vi "Stop.vi"(8 "error in (no error)":errorcluster, 11 "RIO_API in":refnum<class "9770 API.lvclass">) -> (0 "error out":errorcluster, 3 "RIO_API out":refnum<class "9770 API.lvclass">)   [LabVIEW 2017, in "9770 API.lvclass"]
uses:
  <vilib>/addons/InsightCM/Devices/Shared/Emsa/Emsa9770API/9770 API.lvclass
  <vilib>/addons/InsightCM/Devices/Shared/Emsa/Emsa9770API/9770 API.lvclass/9770 API.ctl
  <vilib>/Utility/error.llb/Error Cluster From Error Code.vi
  <vilib>/rvi/errors/niLvFpgaAdjustHostInterfaceError.vi
  <vilib>/ErrorRing/Error Ring.xnode
  <vilib>/rvi/interface/nirviReadWriteControl/nirviReadWriteControl.xnode
  <vilib>/addons/InsightCM/Devices/Shared/Emsa/Emsa9770API/controls/FPGATypeDef.ctl
  NiFpgaLv.dll
  <vilib>/rvi/interface/Simulation/niFpgaSimulationCallBeginRW.vi
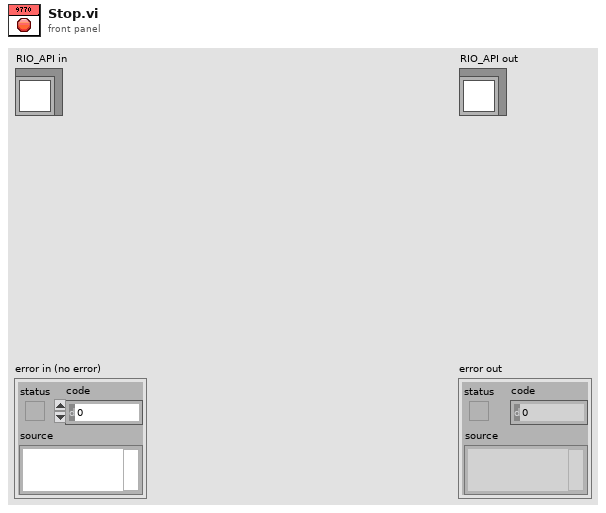
[diagram p1: front panel]
types:
  T1 = typedef "9770 API.lvclass/FPGATypeDef.ctl" = refnum<k20>
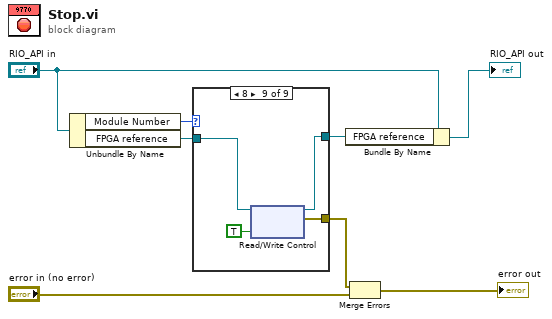
[diagram p0: block diagram]
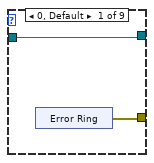
[diagram p2: hidden frame]
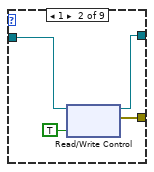
[diagram p3: hidden frame]
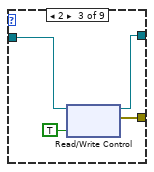
[diagram p4: hidden frame]
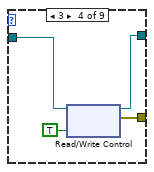
[diagram p5: hidden frame]
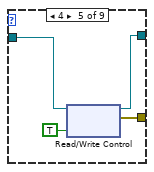
[diagram p6: hidden frame]
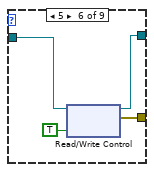
[diagram p7: hidden frame]
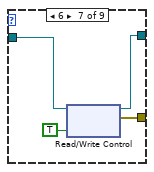
[diagram p8: hidden frame]
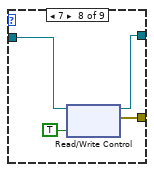
[diagram p9: hidden frame]
diagram:
  n1 = Unbundle By Name("RIO_API in") -> ("Module Number"=w6:u32, "FPGA reference"=w5:T1)
  n2 = case shown="8" w6 {
    tunnel: [w9 w15 w19 w23 w27 w31 w35 w39 w43] -> w4
    tunnel: w5 -> [w10 w14 w18 w22 w26 w30 w34 w38 w42]
    tunnel: [w10 w13 w17 w21 w25 w29 w33 w37 w41] -> w2
    frame 0, Default {
      n3 = xnode "Error Ring"() -> ("error out"=w9:errorcluster)
    }
    frame 1 {
      n4 = xnode "Read/Write Control"("FPGA VI Reference In"=w14, "Stop 1"=TRUE ("Start 1")) -> ("FPGA VI Reference Out"=w13:T1, "error out"=w15:errorcluster)  [unwired: 1 in]
    }
    frame 2 {
      n5 = xnode "Read/Write Control"("FPGA VI Reference In"=w18, "Stop 2"=TRUE ("Start 1")) -> ("FPGA VI Reference Out"=w17:T1, "error out"=w19:errorcluster)  [unwired: 1 in]
    }
    frame 3 {
      n6 = xnode "Read/Write Control"("FPGA VI Reference In"=w22, "Stop 3"=TRUE ("Start 1")) -> ("FPGA VI Reference Out"=w21:T1, "error out"=w23:errorcluster)  [unwired: 1 in]
    }
    frame 4 {
      n7 = xnode "Read/Write Control"("FPGA VI Reference In"=w26, "Stop 4"=TRUE ("Start 1")) -> ("FPGA VI Reference Out"=w25:T1, "error out"=w27:errorcluster)  [unwired: 1 in]
    }
    frame 5 {
      n8 = xnode "Read/Write Control"("FPGA VI Reference In"=w30, "Stop 5"=TRUE ("Start 1")) -> ("FPGA VI Reference Out"=w29:T1, "error out"=w31:errorcluster)  [unwired: 1 in]
    }
    frame 6 {
      n9 = xnode "Read/Write Control"("FPGA VI Reference In"=w34, "Stop 6"=TRUE ("Start 1")) -> ("FPGA VI Reference Out"=w33:T1, "error out"=w35:errorcluster)  [unwired: 1 in]
    }
    frame 7 {
      n10 = xnode "Read/Write Control"("FPGA VI Reference In"=w38, "Stop 7"=TRUE ("Start 1")) -> ("FPGA VI Reference Out"=w37:T1, "error out"=w39:errorcluster)  [unwired: 1 in]
    }
    frame 8 {
      n11 = xnode "Read/Write Control"("FPGA VI Reference In"=w42, "Stop 8"=TRUE ("Start 1")) -> ("FPGA VI Reference Out"=w41:T1, "error out"=w43:errorcluster)  [unwired: 1 in]
    }
  }
  n12 = Bundle By Name(cluster="RIO_API in", "FPGA reference"=w2) -> (→"RIO_API out":refnum<class "9770 API.lvclass">)
  n13 = Merge Errors(w4, "error in (no error)") -> (→"error out":errorcluster)
